vi "Drop_DecodeIncomingPacket.vi"   [LabVIEW 2013]
uses:
  ControlPacket/ControlPacket.lvclass
  MQTT_311/MQTTVersion.lvclass
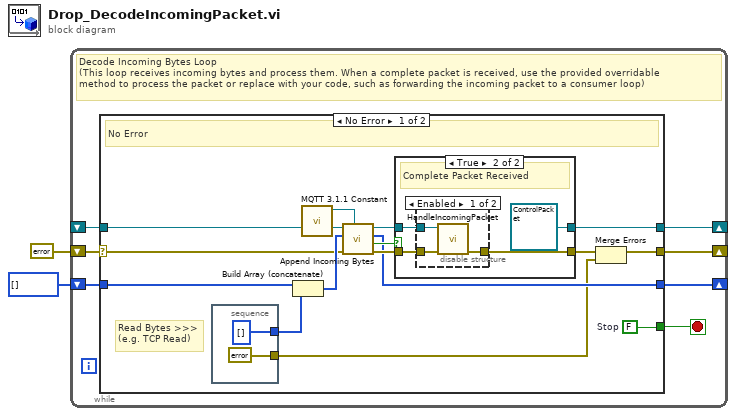
[diagram p0: block diagram]
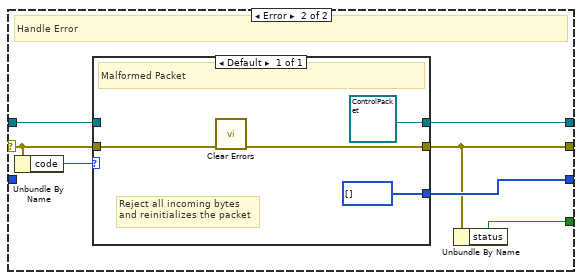
[diagram p4: hidden frame]
diagram:
  n1 = while {
    shift-right: [w7] -> _
    shift-left: u8[] [] ("Remaining Packets") -> [w6]
    shift-right: [w5] -> _
    shift-left: errorcluster {"status"=FALSE, "code"=0, "source"=""} ("error out") -> [w4]
    shift-right: [w8] -> _
    shift-left: _ -> [w9]
    stop <- w3 stop-if-true
    # "Decode Incoming Bytes Loop\n(This loop receives incoming bytes and process them. When a complete packet is received, use the provided overridable \nmethod to process the packet or replace with your code, such as forwarding the incoming packet to a consumer loop)"
    n2 = case shown="No Error" w4 {
      selector: w4 -> [w11 w40]
      tunnel: w9 -> [w24 w38]
      tunnel: [w18 w42] -> w8
      tunnel: [w16 w41] -> w7
      tunnel: w6 -> [w15 _]
      tunnel: [w12 w37] -> w5
      tunnel: [w10 w36] -> w3
      frame No Error {
        w10 = FALSE  # Stop
        # "Read Bytes >>>\n(e.g. TCP Read)"
        # "No Error"
        n3 = stacked-sequence {
          tunnel: [u8[] [] ("Remaining Packets")] -> w23
          tunnel: [errorcluster {"status"=FALSE, "code"=0, "source"=""} ("error out")] -> w14
          frame #0 {
          }
        }
        n4 = Build Array (concatenate)(w15, w23) -> (w22:u8[])
        n5 = call "MQTT 3.1.1 Constant.vi"() -> ("MQTT 3.1.1"=w21:refnum<class "MQTTVersion.lvclass">)  [unwired: 11 in]
        n6 = call "Append Incoming Bytes.vi"("MQTT Version (3.1.1)"=w21, "error in (no error)"=w11, "Incoming Packets"=w22, "Incomplete ControlPacket"=w24) -> ("error out"=w17:errorcluster, "Complete Packet"=w20:bool, "Remaining Packets"=w16:u8[], "ControlPacket"=w19:refnum<class "ControlPacket.lvclass">)  [unwired: 4 in]
        n7 = case shown="True" w20 {
          tunnel: w19 -> [w25 w28]
          tunnel: [w25 refnum<class "ControlPacket.lvclass"> refnum ("ControlPacket")] -> w18
          tunnel: [_ w27] -> w13
          tunnel: w17 -> [_ w26]
          frame False {
            # "None or Partial Packet received"
          }
          frame True {
            # "Complete Packet Received"
            n8 = disable-structure shown="Enabled" {
              disable-tunnel: w28 -> [w32 _]
              disable-tunnel: [w31 w33] -> w27
              disable-tunnel: w26 -> [w30 w33]
              frame Enabled {
                n9 = call-dynamic "HandleIncomingPacket.vi"("error in (no error)"=w30, "ControlPacket in"=w32) -> ("error out"=w31:errorcluster)  [unwired: 8 in, 1 out]
              }
              frame Disabled {
                # "your\ncode"
              }
            }
          }
        }
        n10 = Merge Errors(w13, w14) -> (w12:errorcluster)
      }
      frame Error {
        # "Handle Error"
        n11 = Unbundle By Name(w40) -> ("code"=w39:i32)
        n12 = case shown="Default" w39 {
          tunnel: [refnum<class "ControlPacket.lvclass"> refnum ("ControlPacket")] -> w42
          tunnel: w40 -> [w45]
          tunnel: [w44] -> w37
          tunnel: [u8[] [] ("Remaining Packets")] -> w41
          tunnel: w38 -> [_]
          frame Default {
            # "Reject all incoming bytes\nand reinitializes the packet"
            # "Malformed Packet"
            n13 = call <vilib>:"Clear Errors.vi"("error in (no error)"=w45) -> ("error out"=w44:errorcluster)  [unwired: 6 in]
          }
        }
        n14 = Unbundle By Name(w37) -> ("status"=w36:bool)
      }
    }
  }
